vi "Clear Trigger.vi"(6 "Parent VI":refnum<vi>, 8 "error in (no error)":errorcluster) -> (0 "error out":errorcluster)   [LabVIEW 2015, in "FPGA Addon Engine.lvlib" / "Inline Async API.lvlib"]
uses:
  Inline Async API.lvlib
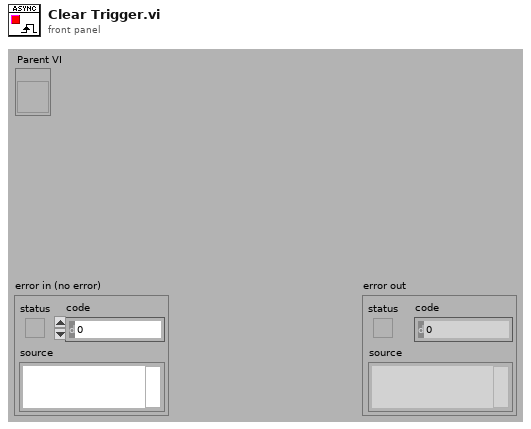
[diagram p1: front panel]
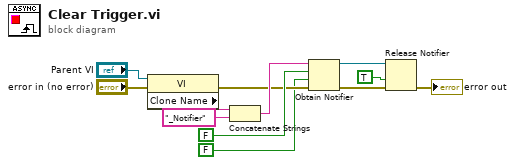
[diagram p0: block diagram]
diagram:
  n1 = property class="VI"(reference="Parent VI", error in="error in (no error)") -> (error out=w6:errorcluster, "Clone Name"=w10:string)  [unwired: 1 out]
  n2 = Concatenate Strings(w10, "_Notifier" ("name (unnamed)")) -> (w8:string)
  n3 = Obtain Notifier(name (unnamed)=w8, notification data type=FALSE, create if not found? (T)=FALSE, error in (no error)=w6) -> (notifier out=w1:refnum<notifier>, error out=w3:errorcluster)  [unwired: 1 out]
  n4 = Release Notifier(notifier=w1, force destroy? (F)=TRUE ("notification"), error in (no error)=w3) -> (error out=→"error out":errorcluster)  [unwired: 2 out]
